vi "append_to_log.vi"(5 "data_type":T1, 7 "dims":T2, 8 "error in (no error)":errorcluster, 9 "Location":string, 10 "Data":variant, 11 "hdf5_photon_record_log in":refnum<class "hdf5_photon_record_log.lvclass">) -> (0 "error out":errorcluster, 3 "hdf5_photon_record_log out":refnum<class "hdf5_photon_record_log.lvclass">)   [LabVIEW 2015, in "hdf5_photon_record_log.lvclass"]
uses:
  hdf5_photon_record_log.lvclass
  Data Logger Class/data_dimensionality.ctl
  Data Logger Class/logger_data_types.ctl
  Picoquant_generic/picoquant_data_tdef.ctl
  hdf5_photon_record_log.lvclass/hdf5_photon_record_log.ctl
  <vilib>/UPVI/lvhdf5/dataset.llb/Append Element(s) to Dataset (Variant).vi
  <vilib>/UPVI/lvhdf5/dataset.llb/Append Element(s) to Dataset.xnode
  <vilib>/UPVI/lvhdf5/library.llb/HDF5 Ref.ctl
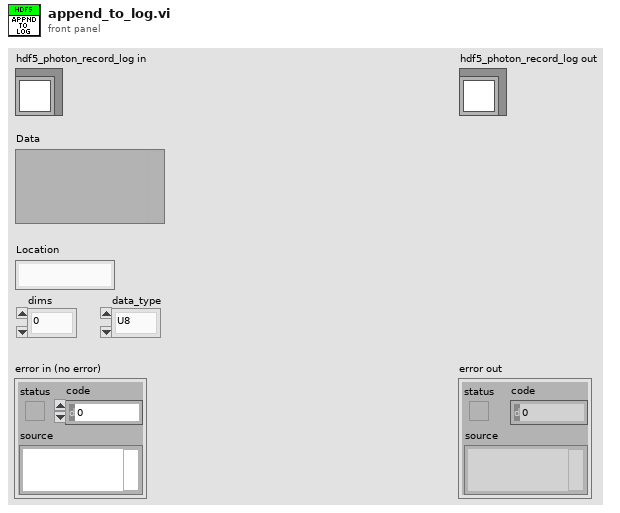
[diagram p1: front panel]
types:
  T1 = typedef "logger_data_types.ctl" = enum16{"U8", "I8", "U16", "I16", "U32", "I32", "DBL", "String"}
  T2 = typedef "data_dimensionality.ctl" = enum16{"0", "1", "2"}
  T3 = typedef "picoquant_data_tdef.ctl" = cluster{"channels":u8[], "times":u64[], "sync":u64[]}
  T4 = typedef "HDF5 Ref.ctl" = refnum<k1>
  T5 = typedef "hpanel_acq_modes.ctl" = u16
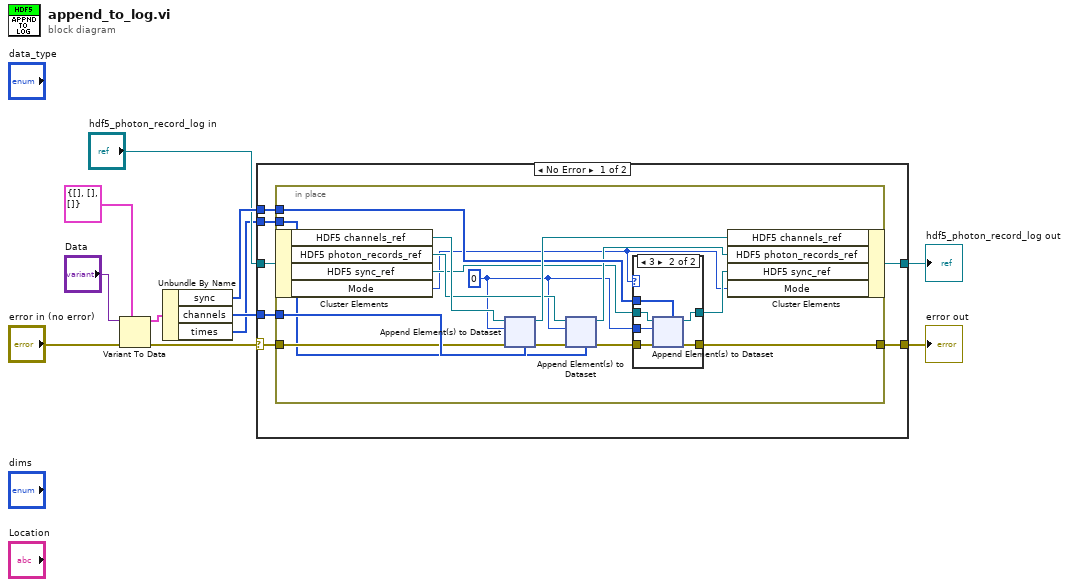
[diagram p0: block diagram]
diagram:
  n1 = Variant To Data(error in="error in (no error)", type=T3 {"channels"=[], "times"=[], "sync"=[]} ("data 2"), Variant="Data") -> (data=w7:T3, error out=w9:errorcluster)
  n2 = Unbundle By Name(w7) -> ("sync"=w6:u64[], "channels"=w2:u8[], "times"=w1:u64[])
  n3 = case shown="No Error" w9 {
    selector: w9 -> [w16 w67]
    tunnel: "hdf5_photon_record_log in" -> [w18 w66]
    tunnel: w2 -> [w17 _]
    tunnel: [w15 w67] -> w3
    tunnel: w1 -> [w14 _]
    tunnel: w6 -> [w13 _]
    tunnel: [w12 w66] -> w4
    frame No Error {
      n4 = in-place {
        in-place-border: w17 -> [w31]
        in-place-border: w16 -> [w28]
        in-place-border: [w27] -> w15
        in-place-border: w14 -> [w20]
        in-place-border: w13 -> [w26]
        w21 = 0 ("Dimension to Extend (0)")
        n5 = in-place-cluster #1(w18) -> ("HDF5 channels_ref"=w33:T4, "HDF5 photon_records_ref"=w25:T4, "HDF5 sync_ref"=w23:T4, "Mode"=w19:T5)
        n6 = xnode "Append Element(s) to Dataset"("Dimension to Extend (0)"=w21, "HDF5 Dataset Ref"=w33, "error in (no error)"=w28, "Data Element(s)"=w31) -> ("HDF5 Dataset out"=w32:T4, "error out"=w30:errorcluster)  [unwired: 2 out]
        n7 = xnode "Append Element(s) to Dataset"("Dimension to Extend (0)"=w21, "HDF5 Dataset Ref"=w25, "error in (no error)"=w30, "Data Element(s)"=w20) -> ("HDF5 Dataset out"=w24:T4, "error out"=w29:errorcluster)  [unwired: 2 out]
        n8 = case shown="3" w19 {
          tunnel: w29 -> [w35 w41]
          tunnel: [w35 w40] -> w27
          tunnel: w26 -> [_ w39]
          tunnel: w23 -> [w34 w38]
          tunnel: [w34 w37] -> w22
          tunnel: w21 -> [_ w36]
          frame 2, Default {
          }
          frame 3 {
            n9 = xnode "Append Element(s) to Dataset"("Dimension to Extend (0)"=w36, "HDF5 Dataset Ref"=w38, "error in (no error)"=w41, "Data Element(s)"=w39) -> ("HDF5 Dataset out"=w37:T4, "error out"=w40:errorcluster)  [unwired: 2 out]
          }
        }
        n10 = in-place-cluster #1("HDF5 channels_ref"=w32, "HDF5 photon_records_ref"=w24, "HDF5 sync_ref"=w22, "Mode"=w19) -> (w12:refnum<class "hdf5_photon_record_log.lvclass">)
      }
    }
    frame Error {
    }
  }
  "error out" <- w3
  "hdf5_photon_record_log out" <- w4
